vi "Read Remote Interlock.vi"(0 "VISA resource name":refnum<visa-resource-name>, 11 "error in (no error)":errorcluster) -> (4 "VISA resource name out":refnum<visa-resource-name>, 6 "Remote Interlock":bool, 15 "error out":errorcluster)   [LabVIEW 2020, in "eec EST 300.lvlib"]
doc: "RI?\nRead the remote Interlock input signal. The interlock is a safety contact that prevents a test from running when in the open state \"1\". When the interlock is shorted a state of \"0\" will allow a test to execute. The interlock requires a constant state of zero till test completion."
uses:
  <instrlib>/eec EST 300/eec EST 300.lvlib
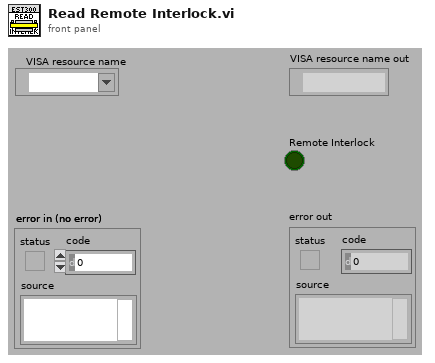
[diagram p1: front panel]
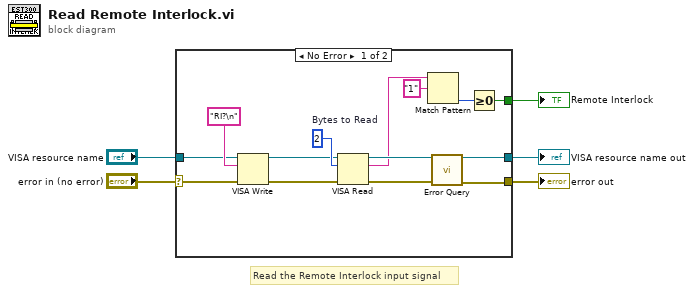
[diagram p0: block diagram]
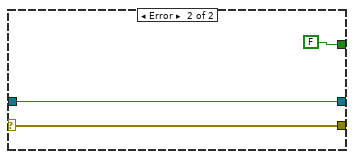
[diagram p2: hidden frame]
diagram:
  # "Read the Remote Interlock input signal"
  n1 = case shown="No Error" "error in (no error)" {
    selector: "error in (no error)" -> [w16 w22]
    tunnel: [w18 w22] -> w4
    tunnel: [w19 w21] -> w2
    tunnel: "VISA resource name" -> [w15 w21]
    tunnel: [w6 FALSE ("Boolean Response")] -> w1
    frame No Error {
      w14 = u32 2  # Bytes to Read
      n2 = VISA Write(VISA resource name=w15, write buffer="RI?\n" ("\"False\" Command"), error in (no error)=w16) -> (VISA resource name out=w11:refnum<visa-resource-name>, error out=w10:errorcluster)  [unwired: 1 out]
      n3 = VISA Read(VISA resource name=w11, byte count=w14, error in (no error)=w10) -> (VISA resource name out=w13:refnum<visa-resource-name>, read buffer=w7:string, error out=w12:errorcluster)  [unwired: 1 out]
      n4 = Match Pattern(string=w7, regular expression="1") -> (offset past match=w8:i32)  [unwired: 1 in, 3 out]
      n5 = call <instrlib>:"Error Query.vi"("VISA resource name"=w13, "error in (no error)"=w12) -> ("VISA resource name out"=w19:refnum<visa-resource-name>, "error out"=w18:errorcluster)  [unwired: 10 in, 2 out]
      n6 = Greater Or Equal To 0?(x=w8) -> (x >= 0?=w6:bool)
    }
    frame Error {
    }
  }
  "error out" <- w4
  "VISA resource name out" <- w2
  "Remote Interlock" <- w1
